vi "Set Pins Infos.vi"(0 "Display State In":T3, 7 "Pin Info Array":T1, 9 "Container State":T4, 11 "error in (no error)":errorcluster) -> (4 "Display State Out":T3, 15 "error out":errorcluster)   [LabVIEW 2021, in "myRIO MSP.xctl"]
uses:
  <vilib>/myRIO/Common/Instrument Driver Framework/Utilities/xctls/myRIO MSP/myRIO MSP.xctl
  <vilib>/_xctls/Container State.ctl
  <vilib>/myRIO/Common/Instrument Driver Framework/Utilities/xctls/myRIO MSP/State.ctl
  <vilib>/myRIO/Common/Instrument Driver Framework/Utilities/xctls/utilities/typedefs/myRIOXC Pin Info Array.ctl
  <vilib>/myRIO/Common/Instrument Driver Framework/Utilities/xctls/utilities/typedefs/myRIOXC Pin Info.ctl
  <vilib>/myRIO/Common/Instrument Driver Framework/Utilities/xctls/utilities/vis/myRIOXC Set Pin Info.vi
  <vilib>/_xctls/XControlSupport.lvlib
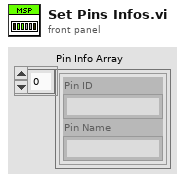
[diagram p1: front panel]
types:
  T1 = typedef "myRIOXC Pin Info Array.ctl" = T2[]
  T2 = typedef "myRIOXC Pin Info.ctl" = cluster{"Pin ID":string, "Pin Name":string}
  T3 = typedef "myRIO MSP.xctl/State.ctl" = cluster{"Pin Disabled?":enum8{"Enabled", "Disabled", "Disabled and Grayed Out"}[], "Pin Name":string[]}
  T4 = typedef "XControlSupport.lvlib/Container State.ctl" = cluster{"Indicator?":bool, "Run Mode?":bool, " Refnum":refnum<vi>}
  T5 = typedef "myRIOXC Display State.ctl" = cluster{"Pin Disabled?":enum8{"Enabled", "Disabled", "Disabled and Grayed Out"}[], "Pin Name":string[]}
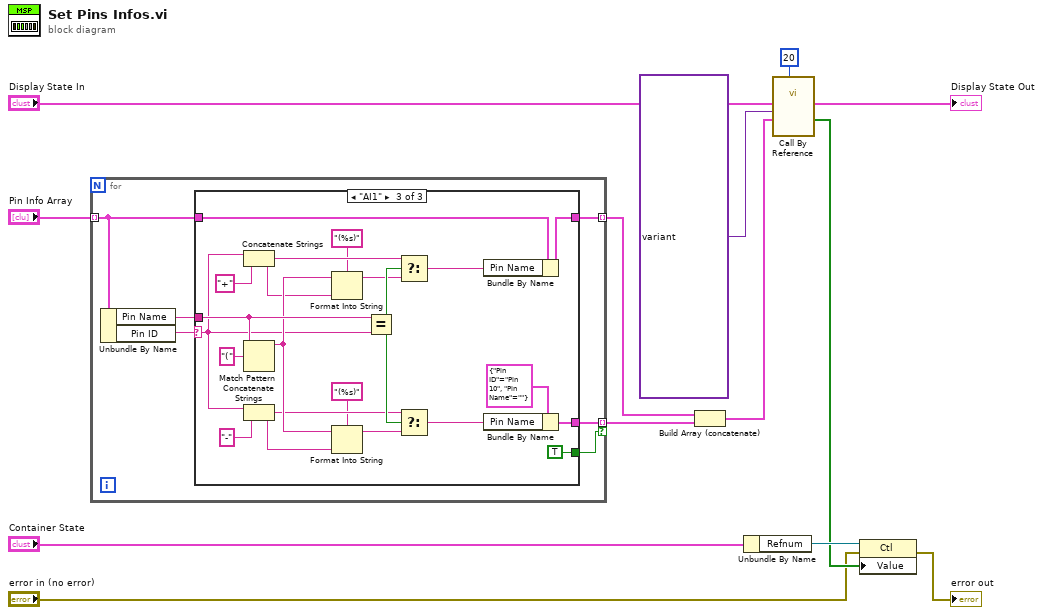
[diagram p0: block diagram]
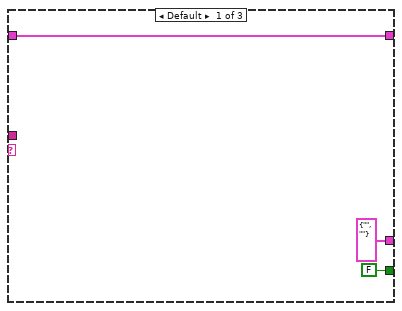
[diagram p2: hidden frame]
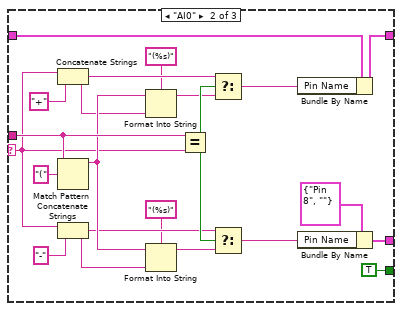
[diagram p3: hidden frame]
diagram:
  n1 = for {
    tunnel: "Pin Info Array" -> [w19] mode=indexing
    tunnel: [w18] -> w3 mode=indexing
    tunnel: [w17] -> w2 mode=indexing if=w14
    n2 = Unbundle By Name(w19) -> ("Pin Name"=w16:string, "Pin ID"=w15:string)
    n3 = case shown="\"AI1\"" w15 {
      selector: w15 -> [_ w24 w44]
      tunnel: w19 -> [w22 w42 w62]
      tunnel: [w22 w41 w61] -> w18
      tunnel: [T2 {"Pin ID"="", "Pin Name"=""} ("Cluster") w39 w59] -> w17
      tunnel: w16 -> [_ w35 w55]
      tunnel: [FALSE TRUE TRUE] -> w14
      frame Default {
      }
      frame "AI0" {
        n4 = Concatenate Strings(w24, "+" ("string")) -> (w30:string)
        n5 = Match Pattern(string=w35, regular expression="(") -> (before substring=w31:string)  [unwired: 1 in, 3 out]
        n6 = Concatenate Strings(w24, "-" ("string")) -> (w29:string)
        n7 = Format Into String(format string="(%s)", initial string=w31, w30) -> (resulting string=w33:string)  [unwired: 1 in, 1 out]
        n8 = Format Into String(format string="(%s)", initial string=w31, w29) -> (resulting string=w32:string)  [unwired: 1 in, 1 out]
        n9 = Equal?(x=w35, y=w24) -> (x = y?=w38:bool)
        n10 = Select(t=w30, s=w38, f=w33) -> (s? t:f=w25:string)
        n11 = Select(t=w29, s=w38, f=w32) -> (s? t:f=w26:string)
        n12 = Bundle By Name(cluster=w42, "Pin Name"=w25) -> (w41:T2)
        n13 = Bundle By Name(cluster=T2 {"Pin ID"="Pin 8", "Pin Name"=""} ("Cluster"), "Pin Name"=w26) -> (w39:T2)
      }
      frame "AI1" {
        n14 = Concatenate Strings(w44, "+" ("string")) -> (w50:string)
        n15 = Match Pattern(string=w55, regular expression="(") -> (before substring=w51:string)  [unwired: 1 in, 3 out]
        n16 = Concatenate Strings(w44, "-" ("string")) -> (w49:string)
        n17 = Format Into String(format string="(%s)", initial string=w51, w50) -> (resulting string=w53:string)  [unwired: 1 in, 1 out]
        n18 = Format Into String(format string="(%s)", initial string=w51, w49) -> (resulting string=w52:string)  [unwired: 1 in, 1 out]
        n19 = Equal?(x=w55, y=w44) -> (x = y?=w58:bool)
        n20 = Select(t=w50, s=w58, f=w53) -> (s? t:f=w45:string)
        n21 = Select(t=w49, s=w58, f=w52) -> (s? t:f=w46:string)
        n22 = Bundle By Name(cluster=w62, "Pin Name"=w45) -> (w61:T2)
        n23 = Bundle By Name(cluster=T2 {"Pin ID"="Pin 10", "Pin Name"=""} ("Cluster"), "Pin Name"=w46) -> (w59:T2)
      }
    }
  }
  n24 = Build Array (concatenate)(w3, w2) -> (w5:T2[])
  n25 = Unbundle By Name("Container State") -> ("Refnum"=w9:refnum<vi>)
  n26 = call-by-ref "?"("Size"=20, "Pin Name Array"=w5, "Pin ID Map"=variant("AI0"=variant(i32 6), "AI1"=variant(i32 8), "AO0"=variant(i32 3), "AO1"=variant(i32 4), "DIO0"=variant(i32 10), "DIO1"=variant(i32 11), "DIO2"=variant(i32 12), "DIO3"=variant(i32 13), "DIO4"=variant(i32 14), "DIO5"=variant(i32 15), "DIO6"=variant(i32 16), "DIO7"=variant(i32 17), "Pin 1"=variant(i32 0), "Pin 10"=variant(i32 9), "Pin 19"=variant(i32 18), "Pin 2"=variant(i32 1), "Pin 20"=variant(i32 19), "Pin 3"=variant(i32 2), "Pin 6"=variant(i32 5), "Pin 8"=variant(i32 7)) ("myRIO MSP"), "Display State In in"="Display State In") -> ("Data"=w8:bool[], "Display State In out"=→"Display State Out":T5)  [unwired: 8 in, 2 out]
  n27 = property class="Ctl"(reference=w9, error in="error in (no error)", "Value"=w8) -> (error out=→"error out":errorcluster)  [unwired: 1 out]
